vi "struct_ads_vol_T_pwpsatRho.vi"(5 "Density of adsorpt in kg/m3 (Input)":dbl, 7 "Saturation pressure in Pa (Input)":dbl, 8 "Error (Input)":errorcluster, 9 "Loading in kg/kg (Input)":dbl, 10 "Pressure in Pa (Input)":dbl, 11 "Reference working pair (Input)":i64) -> (0 "Error (Output)":errorcluster caption="Error(Output)", 3 "Equilibrium temperature in K (Output)":dbl)   [LabVIEW 2017]
doc: "ads_vol_T_pwpsatRho:\n * --------------------\n *\n * Calculates equilibrium temperature T in K depending on equilibrium pressure\n * in Pa, equilibrium loading w in kg/kg, saturation pressure p_Sat in Pa and\n * density of adsorpt rho in kg/m³.\n *\n * Parameters:\n * -----------\n * double p_Pa:\n * Equilibrium pressure in Pa.\n * double w_kgkg:\n * Equilibrium loading in kg/kg.\n * double p_sat_Pa:\n * Saturation pressure in Pa.\n * double rho_kgm3:\n * Density of adsorpt in kg/m³.\n * struct *WorkingPair:\n * Pointer of WorkingPair-struct.\n *\n * Returns:\n * --------\n * double:\n * Equilibrium temperature in K.\n *\n * Remarks:\n * --------\n * This function is only valid for isotherm models based on the volumetric\n * approach.\n * Uses internal equations of states to calculate vapor pressure, saturated\n * liquid density of adsorpt, derivative of vapor pressure wrt. temperature\n * and derivative of saturated liquid density of adsorpt wrt. temperature. If\n * equation of states are not implemented for refrigerant, function returns -1\n * and throws warning. If user want to use his own equation of states, this\n * function cannot be used and determination of root to calculate T must\n * be implemented by user.\n *\n * History:\n * --------\n * 07/13/2021, by Jannik Driesel (supervised by Mirko Engelpracht):\n * First implementation."
uses:
  data/win32bit/libsorpPropLib.dll
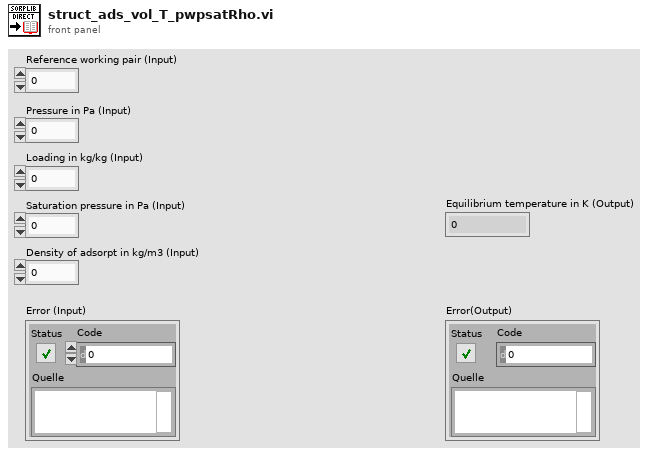
[diagram p1: front panel]
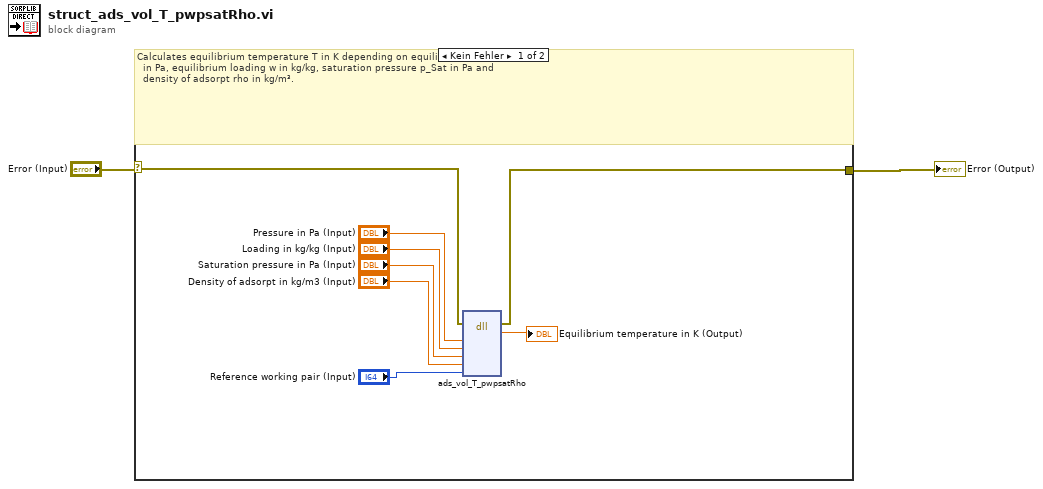
[diagram p0: block diagram]
diagram:
  n1 = case shown="Kein Fehler" "Error (Input)" {
    selector: "Error (Input)" -> [w9 w11]
    tunnel: [w8 w11] -> w1
    frame No Error {
      # "Calculates equilibrium temperature T in K depending on equilibrium pressure\n  in Pa, equilibrium loading w in kg/kg, saturation pressure p_Sat in Pa and\n  density of adsorpt rho in kg/m³."
      n2 = dll-call lib="D:/Driesel/SorpLibLocal/LabVIEW_wrapper/data/win32bit/libsorpPropLib.dll" fn="ads_vol_T_pwpsatRho"(error in=w9, "p_Pa"="Pressure in Pa (Input)", "w_kgkg"="Loading in kg/kg (Input)", "p_sat_Pa"="Saturation pressure in Pa (Input)", "rho_kgm3"="Density of adsorpt in kg/m3 (Input)", "workingPair"="Reference working pair (Input)") -> (error out=w8:errorcluster, "T_K"=→"Equilibrium temperature in K (Output)":dbl)  [unwired: 7 in, 1 out]
    }
    frame Error {
      # "Error - No calculations"
    }
  }
  "Error (Output)" <- w1
